vi "Main.vi"() -> ()   [LabVIEW 2022 SP3]
doc: "Main Program initialize config files, handles user inputs, image acquisition, object detection and image storing. User interface is handled in a state machine sending outputs."
uses:
  controls/State.ctl
  controls/Data.ctl
  <vilib>/userdefined/High Color/IMAQdx.ctl
  <vilib>/vision/Image Controls.llb/IMAQ Image.ctl
  b1a6e15a-21f6-4224-89c9-cebb1e441bce.vi
  4203ab90-da59-4329-829c-edbd02661f10.vi
  <extravilib>/ChannelInstances/Tag-bool/Read With Abort.vi
  <extravilib>/ChannelInstances/Tag-t'Data.ctl'/Read With Abort.vi
  <extravilib>/ChannelInstances/Tag-c(bool,bool)/Read With Abort.vi
  <extravilib>/ChannelInstances/Tag-c(bool,bool)/Write With Abort.vi
  <extravilib>/ChannelInstances/Tag-t'Data.ctl'/Write With Abort.vi
  <extravilib>/ChannelInstances/Tag-bool/Write With Abort.vi
  <extravilib>/ChannelInstances/Tag-c(bool,bool)/Instantiate.vi
  <extravilib>/ChannelInstances/Tag-t'Data.ctl'/Instantiate.vi
  <extravilib>/ChannelInstances/Tag-bool/Instantiate.vi
  <extravilib>/ChannelInstances/Tag-bool/EndpointRead.vi
  <extravilib>/ChannelInstances/Tag-t'Data.ctl'/EndpointRead.vi
  <extravilib>/ChannelInstances/Tag-c(bool,bool)/EndpointRead.vi
  <extravilib>/ChannelInstances/Tag-c(bool,bool)/Endpoint.vi
  <extravilib>/ChannelInstances/Tag-t'Data.ctl'/Endpoint.vi
  <extravilib>/ChannelInstances/Tag-bool/Endpoint.vi
  <extravilib>/ChannelInstances/Tag-bool.lvlib
  <extravilib>/ChannelInstances/Tag-t'Data.ctl'.lvlib
  <extravilib>/ChannelInstances/Tag-c(bool,bool).lvlib
panel:
  out "System Version":string="SRS Software - Version 0.0.0.1-beta"
  out "error out":errorcluster
  out "Overlay_tab":T1(tab)=enum."Connections"
  out "Cam1_Stats":cluster{"Mean_Area":i32, "Img_Count":u32} caption="Camera 1"
  out "Cam2_Stats":cluster{"Mean_Area":i32, "Img_Count":u32} caption="Camera 2"
  out "Sample Number":string="#0000" caption="Sample Name"
  in  "Collection Date":timestamp=timestamp(3501961200 s since 1904-01-01) format="%<%x>T"
  in  "Station":string="Station..." caption="Sample Name"
  in  "Location":string="Location..." caption="Sample Name"
  in  "Latitude":dbl caption="Sample Name" format="%.8g"
  in  "Longitude":dbl caption="Sample Name" format="%.8g"
  in  "Determiner":string="Name..." caption="Sample Name"
  in  "Sex":string="NaN" caption="Sample Name"
  in  "overloadThreshold":i32=5 caption="Overload threshold" min=1
  in  "saveQueueSize":i32=100 caption="Save Buffer Size" min=1
  in  "processQueueSize":i32=200 caption="Process Buffer Size" min=1
  in  "legacyAttributes":bool caption="Legacy Camera Attributes"
  in  "Change Crop":bool
  in  "DetectCrop":dbl=10.0 caption="Movement Detection size" format="%#_g %"
  in  "sampleSizeThreshold":i32=3000 caption="Sample size threshold" min=1
  in  "sampleTimeout":i32=20 caption="New Sample timeout" min=1
  out "Target framerate":i32=50 caption="Target FPS"
  in  "framerateMax":i32=50 caption="Max FPS" min=1
  in  "Exposure Time":dbl=2000.0
  in  "Exposure":enum32{"Item 0", "Item 1", "Item 2", "Item 3"}(radio)=enum."Item 3"
  in  "Aperture":enum32{"Item 0", "Item 1", "Item 2", "Item 3"}(radio)=enum."Item 1"
  in  "Calibration Pictures":bool
  in  "Empty Cuvette":bool
  in  "Manual Close":bool
  out "Current Position":string
  in  "Position":bool
  in  "flushSize":i32=150 caption="Flush Size" min=0 max=1000
  in  "dispenseDuration":i32=60 caption="Dispense Duration" min=20 max=200
  in  "Pump Cycle":bool
  in  "Pump Bottom":bool
  in  "Pump Top":bool
  in  "Pump Terminate":bool
  out "Process buffer":T2(graph)
  out "Save buffer":T2(graph)
  out "Framerate":i32 caption="Current Framerate"
  out "System Serial":string
  in  "Connect Systems":bool
  out "Actuator":bool
  out "Pump":bool
  out "Camera 1":bool
  out "Camera 2":bool
  in  "Override System":bool
  in  "Empty System":bool
  in  "Start System":bool
  out "Errors":errorcluster
  in  "Overlay_Ring":u16(ring)=6 items=["Session Data", "Extended Setup", "Buffer", "Camera", "Dispenser", "Stats", "Connections", "Errors"]
  in  "otherNotes":string caption="Other notes"
  in  "Species Name":string="System Test - Toke" caption="Sample Name"
  out "Ready":bool
  in  "Operator":string="MRJ" caption="Sample Name"
  out "Active":bool
  in  "Start Image Capture":bool
  in  "voucherId":string="#0000" caption="Voucher ID"
  in  "Stop Image Capture":bool
  in  "Empty and Refill":bool
  in  "Close and Refill":bool
  in  "Manual Open":bool
  out "Detection error":errorcluster
  out "Camera 1":T3(plugin-control)
  out "Camera 2":T3(plugin-control)
  out "Camera 1 Binary":T3(plugin-control)
  out "Camera 2 Binary":T3(plugin-control)
  out "Camera 1 Detect":T3(plugin-control)
  out "Camera 2 Detect":T3(plugin-control)
  # "Description:\nData from the last sample for each camera.\n\nMean area\nMean area  from detection algorithm.\n\nImages\nTotal number of images saved."
  # "Detection settings"
  # "Camera/Lens settings"
  # "Hatch Control"
  # "Pump Control"
  # "Connections"
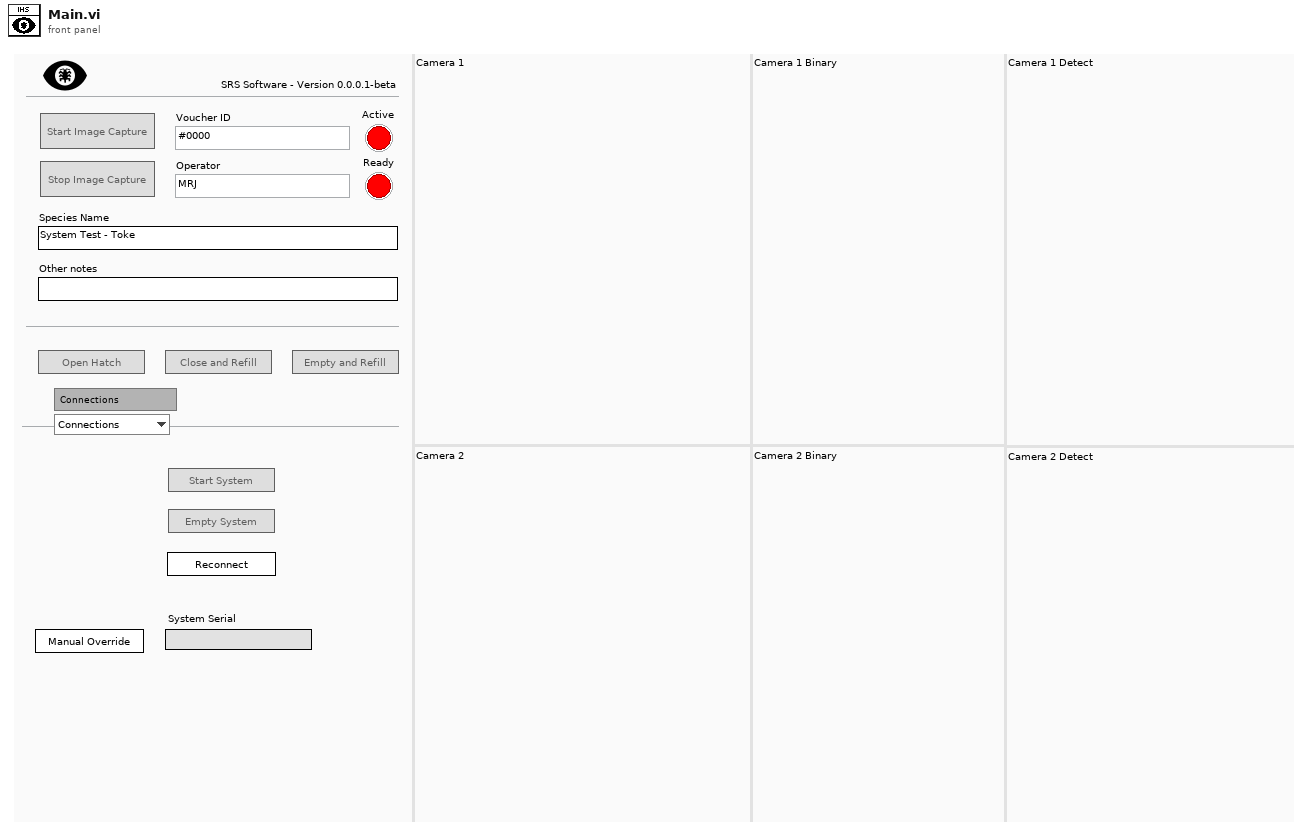
[diagram p1: front panel]
types:
  T1 = enum32{"Session Data", "Extended Setup", "Buffer", "Camera", "Dispenser", "Stats", "Connections", "Errors"}
  T2 = cluster{"# elements in queue":i32, "# elements in queue":i32}
  T3 = typedef "IMAQ Image.ctl" = refnum<image>
  T4 = typedef "Data.ctl" = cluster{"system":cluster{"info":cluster{"menuSelect":u16, "version":u16, "serial":string, "captureActive":bool, "captureBegin":bool, "emptyAndRefill":bool}, "userInfo":cluster{"operatorName":string, "date":timestamp}, "camera":cluster{"exposureTime":i32, "aperture":enum32{"Item 0", "Item 1", "Item 2", "Item 3"}, "framerate":i32, "framerateMax":i32, "legacyAttributes":bool}}, "connections":cluster{"arduino":cluster{"connection":refnum<visa-resource-name>, "status":bool, "openState":bool, "emptyStart":u32}, "pump":cluster{"connection":refnum<visa-resource-name>, "status":bool, "command":string, "dispenseSpeed":i32, "flushSize":i32}, "camera":cluster{"cam1":cluster{"connection":T5, "status":bool}, "cam2":cluster{"connection":T5, "status":bool}}}, "queue":cluster{"process":cluster{"cam1":refnum<queue>, "cam2":refnum<queue>, "queueSize":i32}, "save":cluster{"cam1":refnum<queue>, "cam2":refnum<queue>, "queueSize":i32}, "overloadThreshold":i32}, "imageProcess":cluster{"cam1":cluster{"preAllocation":cluster{"image":T3, "originalDisplay":T3, "originalRgb":T3, "binary":T3, "save":T3, "calibrationFull":T3, "calibrationDetect":T3}, "calibration":cluster{"pathFull":path, "pathDetect":path, "ROI":T6}}, "cam2":cluster{"preAllocation":cluster{"image":T3, "originalDisplay":T3, "originalRgb":T3, "binary":T3, "save":T3, "calibrationFull":T3, "calibrationDetect":T3}, "calibration":cluster{"pathFull":path, "pathDetect":path, "ROI":T6}}, "process":cluster{"planeExtract":T3, "planeSubtract":T3, "cropMask":T3}, "detection":cluster{"sampleTimeout":i32, "sizeThreshold":i32, "detectionRegionPct":dbl}}, "sampleData":cluster{"sampleId":string, "projectId":string, "voucherID":string, "speciesName":string, "collectionDate":timestamp, "sampleStation":string, "location":string, "lat":dbl, "lon":dbl, "determiner":string, "sex":string, "otherNotes":string}, "Session In":T5}
  T5 = typedef "IMAQdx.ctl" = refnum<k21>
  T6 = typedef "IMAQ Rectangle" = cluster{"Left":i32, "Top":i32, "Right":i32, "Bottom":i32, "Rotation":dbl}
  T7 = typedef "State.ctl" = enum16{"Initialize", "Wait for Event", "Position", "Valve Signal", "Extra Flush", "Valve Cycle", "Valve Open", "Valve Close", "Pump Command", "Pump Cycle", "Empty System", "Start System", "Connect Systems", "Start Image Capture", "Stop Image Capture", "Calibration Pictures", "Close and Refill", "Empty and Refill", "Change Light Intensity", "Reconnect", "CursorIdle", "Exit"}
  T8 = enum8{"Enabled", "Disabled", "Disabled and Grayed Out"}
  T9 = cluster{"# elements in queue":i32, "# elements in queue":i32}[]
  T10 = typedef "Tag-t'Data.ctl'.lvlib/))Channel.ctl" = refnum<queue>
  T11 = typedef "Tag-bool.lvlib/))Channel.ctl" = refnum<queue>
  T12 = typedef "Tag-c(bool,bool).lvlib/))Channel.ctl" = refnum<queue>
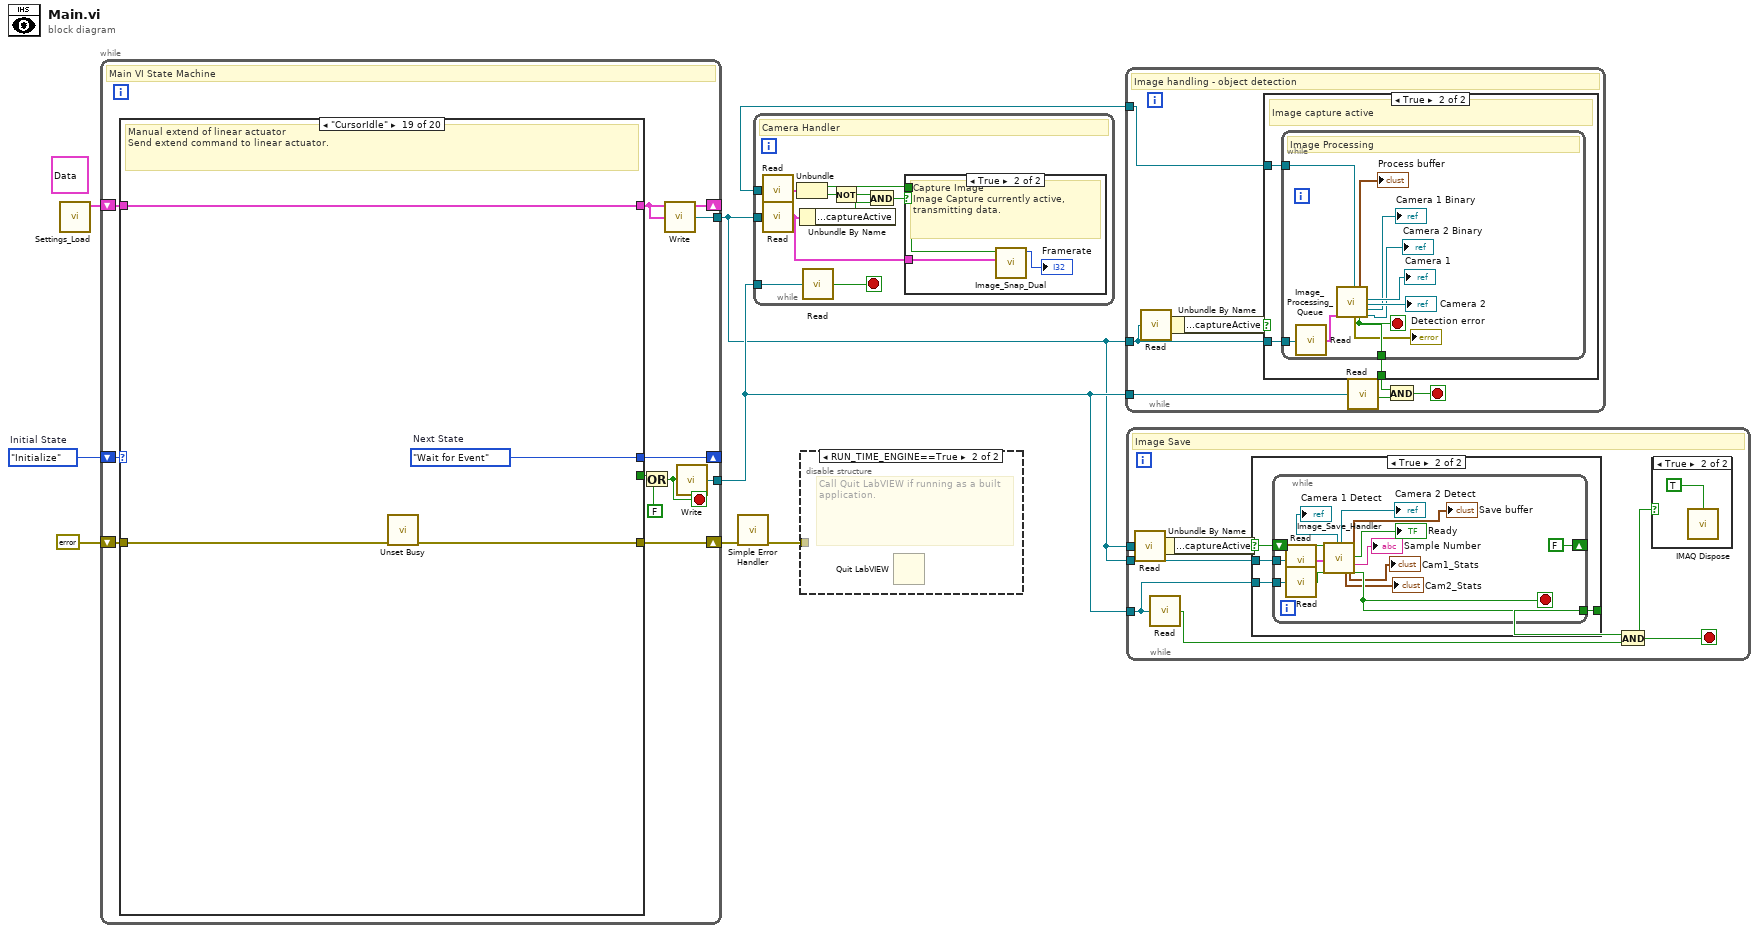
[diagram p0: block diagram]
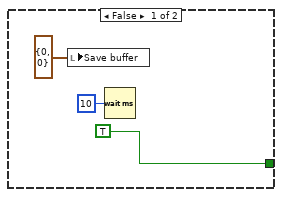
[diagram p3: hidden frame]
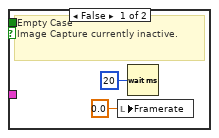
[diagram p4: hidden frame]
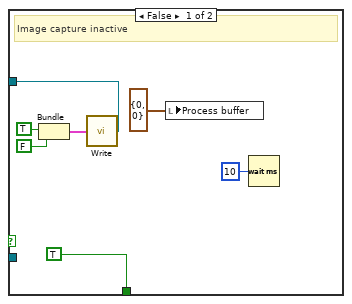
[diagram p5: hidden frame]
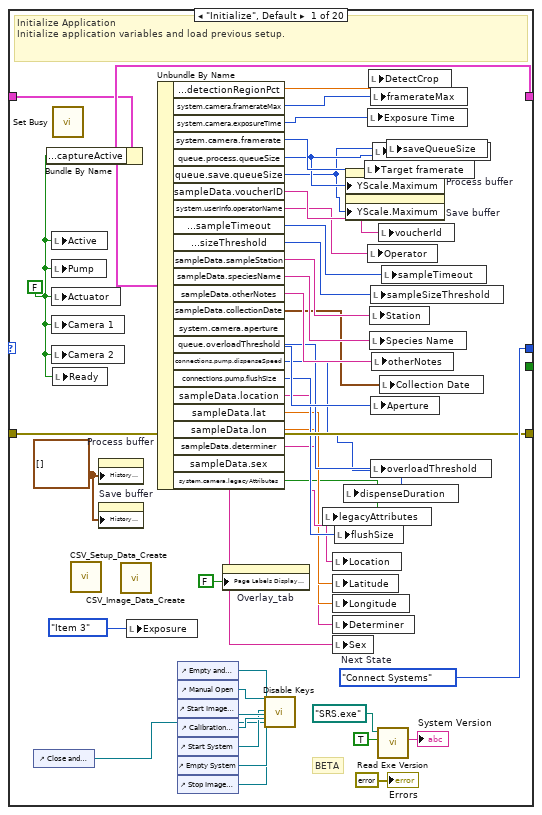
[diagram p7: hidden frame]
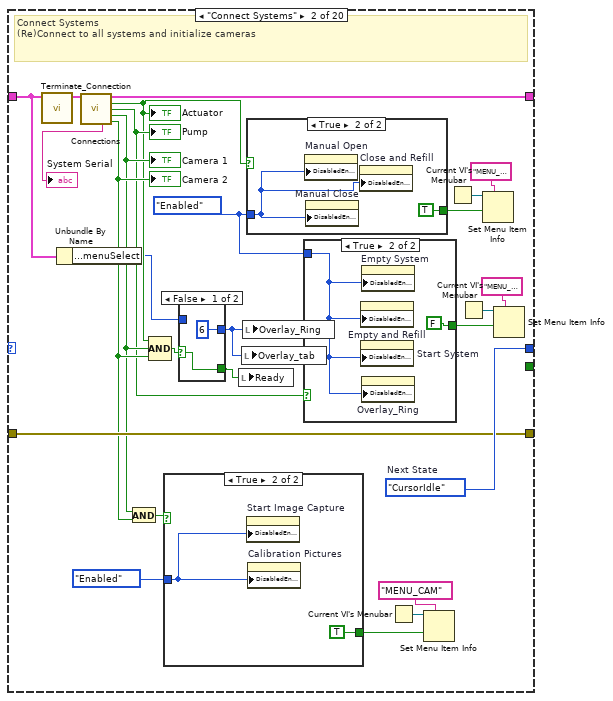
[diagram p8: hidden frame]
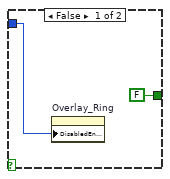
[diagram p10: hidden frame]
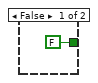
[diagram p11: hidden frame]
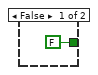
[diagram p12: hidden frame]
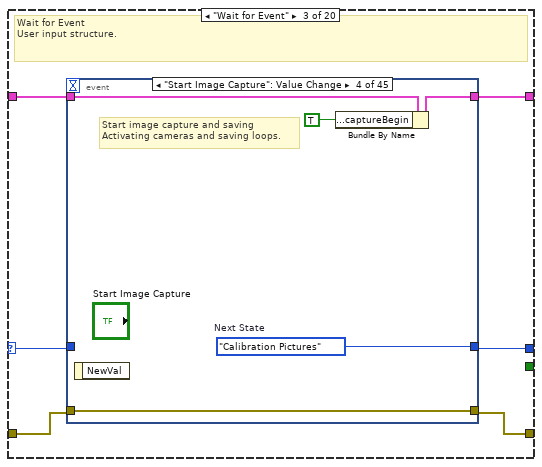
[diagram p13: hidden frame]
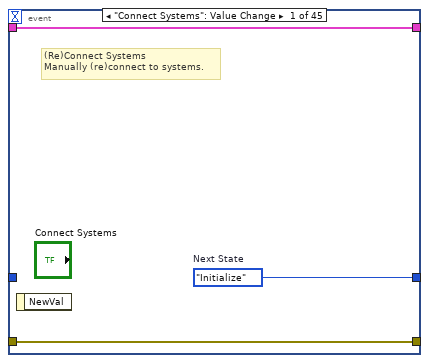
[diagram p14: hidden frame]
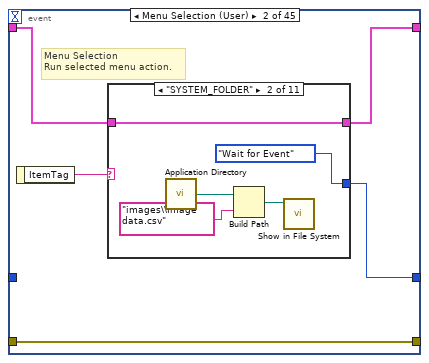
[diagram p15: hidden frame]
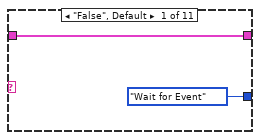
[diagram p16: hidden frame]
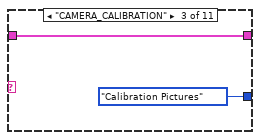
[diagram p17: hidden frame]
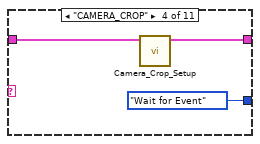
[diagram p18: hidden frame]
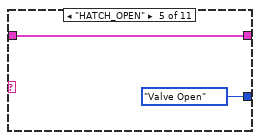
[diagram p19: hidden frame]
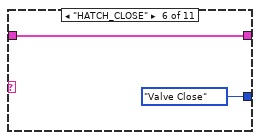
[diagram p20: hidden frame]
diagram:
  (unwired) T4 {"system"={"info"={"menuSelect"=0, "version"=0, "serial"="Test Sample", "captureActive"=FALSE, "captureBegin"=FALSE, "emptyAndRefill"=FALSE}, "userInfo"={"operatorName"="", "date"=timestamp(2713993200 s since 1904-01-01)}, "camera"={"exposureTime"=0, "aperture"=enum."Item 0", "framerate"=0, "framerateMax"=500, "legacyAttributes"=FALSE}}, "connections"={"arduino"={"connection"="", "status"=FALSE, "openState"=FALSE, "emptyStart"=0}, "pump"={"connection"="", "status"=FALSE, "command"="", "dispenseSpeed"=100, "flushSize"=100}, "camera"={"cam1"={"connection"="", "status"=FALSE}, "cam2"={"connection"="", "status"=FALSE}}}, "queue"={"process"={"cam1"=refnum, "cam2"=refnum, "queueSize"=0}, "save"={"cam1"=refnum, "cam2"=refnum, "queueSize"=0}, "overloadThreshold"=0}, "imageProcess"={"cam1"={"preAllocation"={"image"="Station", "originalDisplay"="Station", "originalRgb"="Station", "binary"="Station", "save"="Station", "calibrationFull"=refnum, "calibrationDetect"=refnum}, "calibration"={"pathFull"=path "C:/Users/au540322/Desktop/IHS_Project/images/Debris/Debris_0/Debris_0_2019_06_01-23-32-49-686.PNG", "pathDetect"=path "C:/Users/au540322/Desktop/IHS_Project/images/Debris/Debris_0/Debris_0_2019_06_01-23-32-49-686.PNG", "ROI"={"Left"=0, "Top"=0, "Right"=0, "Bottom"=0, "Rotation"=0.0}}}, "cam2"={"preAllocation"={"image"=refnum, "originalDisplay"=refnum, "originalRgb"=refnum, "binary"=refnum, "save"=refnum, "calibrationFull"=refnum, "calibrationDetect"=refnum}, "calibration"={"pathFull"=path "C:/Users/au540322/Desktop/IHS_Project/images/Debris/Debris_0/Debris_0_2019_06_01-23-32-49-686.PNG", "pathDetect"=path "C:/Users/au540322/Desktop/IHS_Project/images/Debris/Debris_0/Debris_0_2019_06_01-23-32-49-686.PNG", "ROI"={"Left"=0, "Top"=0, "Right"=0, "Bottom"=0, "Rotation"=0.0}}}, "process"={"planeExtract"=refnum, "planeSubtract"=refnum, "cropMask"=refnum}, "detection"={"sampleTimeout"=500, "sizeThreshold"=500, "detectionRegionPct"=0.0}}, "sampleData"={"sampleId"="", "projectId"="", "voucherID"="", "speciesName"="", "collectionDate"=timestamp(2713993200 s since 1904-01-01), "sampleStation"="", "location"="", "lat"=0.0, "lon"=0.0, "determiner"="", "sex"="", "otherNotes"=""}, "Session In"=""} ("Data")
  w8 = State."Initialize"  # Initial State
  n1 = call "Settings_Load.vi"() -> ("value"=w4:T4)  [unwired: 10 in, 1 out]
  n2 = while {
    shift-right: [w18] -> _
    shift-left: w8 -> [w19]
    shift-right: [w16] -> _
    shift-left: w4 -> [w17]
    shift-right: [w13] -> w6
    shift-left: errorcluster {"status"=FALSE, "code"=0, "source"=""} ("error constant") -> [w15]
    tunnel: [w10] -> w3
    tunnel: [w11] -> w2
    stop <- w14 stop-if-true
    # "Main VI State Machine"
    n3 = case shown="\"CursorIdle\"" w19 {
      selector: w19 -> [_ _ w104 _ _ _ _ _ _ _ _ _ _ _ _ _ _ _ _ _]
      tunnel: [w63 w89 w109 w376 w394 w413 w443 w468 w474 w491 w508 w516 w529 w547 w557 w587 w609 w627 w630 w641] -> w18
      tunnel: [_ _ _ _ _ _ _ _ _ _ _ _ _ _ _ _ _ _ _ w640] -> w12
      tunnel: w17 -> [w56 w69 w108 w377 w390 w406 w437 w462 w478 w495 w500 w514 w527 w546 w551 w586 w599 w611 w631 w636]
      tunnel: [w61 w87 w107 w378 w392 w405 w442 w467 w469 w495 w501 w511 w526 w546 w550 w586 w598 w610 w631 w638] -> w16
      tunnel: w15 -> [w62 w88 w106 w379 w393 w412 w432 w457 w477 w492 w506 w519 w531 w542 w554 w583 w606 w624 w629 w634]
      tunnel: [w62 w88 w105 w379 w393 w412 w426 w450 w477 w485 w505 w517 w520 w541 w553 w580 w605 w615 w628 w635] -> w13
      frame "Initialize", Default {
        w55 = T9 [] ("History Data")
        w54 = FALSE ("Pump")
        w63 = State."Connect Systems"  # Next State
        # "BETA"
        # "Initialize Application\nInitialize application variables and load previous setup."
        n4 = control-ref of="Close and Refill"() -> (w39:refnum<vi>)
        n5 = Bundle By Name(cluster=w56, "system.info.captureActive"=w54) -> (w61:T4)
        n6 = local write "Active"(w54) -> ()
        n7 = local write "Pump"(w54) -> ()
        n8 = local write "Actuator"(w54) -> ()
        n9 = local write "Camera 1"(w54) -> ()
        n10 = local write "Camera 2"(w54) -> ()
        n11 = call <vilib>:"Set Busy.vi"() -> ()  [unwired: 10 in, 2 out]
        n12 = local write "Ready"(w54) -> ()
        n13 = call "CSV_Setup_Data_Create.vi"() -> ()  [unwired: 11 in, 1 out]
        n14 = property on="Process buffer" class="WFChart (strict)"("History Data"=w55) -> ()  [unwired: 2 in, 2 out]
        n15 = property on="Save buffer" class="WFChart (strict)"("History Data"=w55) -> ()  [unwired: 2 in, 2 out]
        n16 = call "CSV_Image_Data_Create.vi"() -> ()  [unwired: 12 in]
        n17 = local write "Exposure"(enum32{"Item 0", "Item 1", "Item 2", "Item 3"}."Item 3" ("Exposure")) -> ()
        n18 = Unbundle By Name(w61) -> ("imageProcess.detection.detectionRegionPct"=w36:dbl, "system.camera.framerateMax"=w37:i32, "system.camera.exposureTime"=w60:i32, "system.camera.framerate"=w59:i32, "queue.process.queueSize"=w21:i32, "queue.save.queueSize"=w20:i32, "sampleData.voucherID"=w58:string, "system.userInfo.operatorName"=w57:string, "imageProcess.detection.sampleTimeout"=w53:i32, "imageProcess.detection.sizeThreshold"=w52:i32, "sampleData.sampleStation"=w51:string, "sampleData.speciesName"=w50:string, "sampleData.otherNotes"=w49:string, "sampleData.collectionDate"=w22:timestamp, "system.camera.aperture"=w48:enum32{"Item 0", "Item 1", "Item 2", "Item 3"}, "queue.overloadThreshold"=w47:i32, "connections.pump.dispenseSpeed"=w34:i32, "connections.pump.flushSize"=w35:i32, "sampleData.location"=w33:string, "sampleData.lat"=w32:dbl, "sampleData.lon"=w31:dbl, "sampleData.determiner"=w30:string, "sampleData.sex"=w29:string, "system.camera.legacyAttributes"=w28:bool)
        n19 = control-ref of="Empty and Refill"() -> (w46:refnum<vi>)
        n20 = control-ref of="Manual Open"() -> (w45:refnum<vi>)
        n21 = control-ref of="Start Image Capture"() -> (w43:refnum<vi>)
        n22 = control-ref of="Calibration Pictures"() -> (w44:refnum<vi>)
        n23 = control-ref of="Start System"() -> (w42:refnum<vi>)
        n24 = control-ref of="Empty System"() -> (w41:refnum<vi>)
        n25 = control-ref of="Stop Image Capture"() -> (w40:refnum<vi>)
        n26 = property on="Overlay_tab" class="TabCtl (strict)"("Page Labels Display Visible?"=FALSE) -> ()  [unwired: 2 in, 2 out]
        n27 = call "Disable Keys.vi"("Boolean in"=w45, "Bool Refnum 6"=w46, "Bool Refnum 4"=w40, "Bool Refnum 7"=w42, "Bool Refnum 9"=w43, "Bool Refnum 2"=w44, "Bool Refnum 8"=w39, "Bool Refnum 3"=w41) -> ()  [unwired: 20 in]
        n28 = local write "legacyAttributes"(w28) -> ()
        n29 = local write "Location"(w33) -> ()
        n30 = local write "Latitude"(w32) -> ()
        n31 = local write "Longitude"(w31) -> ()
        n32 = local write "Determiner"(w30) -> ()
        n33 = local write "Sex"(w29) -> ()
        n34 = local write "flushSize"(w35) -> ()
        n35 = local write "dispenseDuration"(w34) -> ()
        n36 = property on="Process buffer" class="WFChart (strict)"("YScale.Maximum"=w21) -> ()  [unwired: 2 in, 2 out]
        n37 = property on="Save buffer" class="WFChart (strict)"("YScale.Maximum"=w20) -> ()  [unwired: 2 in, 2 out]
        n38 = local write "Target framerate"(w59) -> ()
        n39 = local write "Exposure Time"(w60) -> ()
        n40 = local write "Operator"(w57) -> ()
        n41 = local write "DetectCrop"(w36) -> ()
        n42 = local write "Station"(w51) -> ()
        n43 = local write "Species Name"(w50) -> ()
        n44 = local write "framerateMax"(w37) -> ()
        n45 = local write "sampleSizeThreshold"(w52) -> ()
        n46 = local write "Aperture"(w48) -> ()
        n47 = local write "overloadThreshold"(w47) -> ()
        n48 = local write "otherNotes"(w49) -> ()
        n49 = local write "processQueueSize"(w21) -> ()
        n50 = call "Read Exe Version.vi"("beta?"=TRUE, "Application name"=path "SRS.exe") -> ("Title String"=→"System Version":string)  [unwired: 6 in, 3 out]
        n51 = local write "voucherId"(w58) -> ()
        n52 = local write "Collection Date"(w22) -> ()
        n53 = local write "sampleTimeout"(w53) -> ()
        n54 = local write "saveQueueSize"(w20) -> ()
        "Errors" <- errorcluster {"status"=FALSE, "code"=0, "source"=""} ("Calibration Error")
      }
      frame "Connect Systems" {
        w83 = T8."Enabled" ("Disabled")
        w89 = State."CursorIdle"  # Next State
        # "Connect Systems\n(Re)Connect to all systems and initialize cameras"
        n55 = call "Terminate_Connection.vi"("Data"=w69) -> ("Data out"=w86:T4)  [unwired: 9 in, 1 out]
        n56 = Unbundle By Name(w69) -> ("system.info.menuSelect"=w68:u16)
        n57 = call "Connections.vi"("input cluster"=w86) -> ("output cluster"=w87:T4, "Linear Actuator"=w70:bool, "Pump"=w71:bool, "Camear 1"=w72:bool, "System Serial"=→"System Serial":string, "Camera 2"=w73:bool)  [unwired: 9 in]
        "Pump" <- w71
        "Actuator" <- w70
        "Camera 2" <- w73
        "Camera 1" <- w72
        n58 = And(x=w72, y=w73) -> (x .and. y?=w85:bool)
        n59 = Compound Arithmetic op=AND(w70, w72, w73) -> (w67:bool)
        n60 = case shown="True" w85 {
          tunnel: T8."Enabled" ("Disabled") -> [_ w100]
          tunnel: [FALSE ("enabled") TRUE ("enabled")] -> w80
          frame False {
          }
          frame True {
            n61 = property on="Start Image Capture" class="Bool"("DisabledEnum"=w100) -> ()  [unwired: 2 in, 2 out]
            n62 = property on="Calibration Pictures" class="Bool"("DisabledEnum"=w100) -> ()  [unwired: 2 in, 2 out]
          }
        }
        n63 = case shown="False" w67 {
          selector: w67 -> [w90 w92]
          tunnel: w68 -> [_ w93]
          tunnel: [u16 6 ("Overlay_Ring") w93] -> w66
          tunnel: [w90 w92] -> w65
          frame False {
          }
          frame True {
          }
        }
        n64 = local write "Ready"(w65) -> ()
        n65 = local write "Overlay_tab"(w66) -> ()
        n66 = local write "Overlay_Ring"(w66) -> ()
        n67 = case shown="True" w70 {
          tunnel: w83 -> [_ w103]
          tunnel: [FALSE ("enabled") TRUE ("enabled")] -> w77
          frame False {
          }
          frame True {
            n68 = property on="Manual Open" class="Bool"("DisabledEnum"=w103) -> ()  [unwired: 2 in, 2 out]
            n69 = property on="Manual Close" class="Bool"("DisabledEnum"=w103) -> ()  [unwired: 2 in, 2 out]
            n70 = property on="Close and Refill" class="Bool"("DisabledEnum"=w103) -> ()  [unwired: 2 in, 2 out]
          }
        }
        n71 = case shown="True" w71 {
          tunnel: w83 -> [w95 w97]
          tunnel: [FALSE ("enabled") FALSE ("enabled")] -> w74
          frame False {
            n72 = property on="Overlay_Ring" class="Ring (strict)"("DisabledEnum"=w95) -> ()  [unwired: 2 in, 2 out]
          }
          frame True {
            n73 = property on="Empty and Refill" class="Bool"("DisabledEnum"=w97) -> ()  [unwired: 2 in, 2 out]
            n74 = property on="Start System" class="Bool"("DisabledEnum"=w97) -> ()  [unwired: 2 in, 2 out]
            n75 = property on="Empty System" class="Bool"("DisabledEnum"=w97) -> ()  [unwired: 2 in, 2 out]
            n76 = property on="Overlay_Ring" class="Ring (strict)"("DisabledEnum"=w97) -> ()  [unwired: 2 in, 2 out]
          }
        }
        n77 = Current VI's Menubar() -> (w82:refnum<k9>)
        n78 = Set Menu Item Info(7:"MENU_CAM" ("item tag"), 9:w80, 11:w82) -> ()  [unwired: 4 in, 2 out]
        n79 = Current VI's Menubar() -> (w78:refnum<k9>)
        n80 = Current VI's Menubar() -> (w76:refnum<k9>)
        n81 = Set Menu Item Info(7:"MENU_HATCH" ("item tag"), 9:w77, 11:w78) -> ()  [unwired: 4 in, 2 out]
        n82 = Set Menu Item Info(7:"MENU_HATCH" ("item tag"), 9:w74, 11:w76) -> ()  [unwired: 4 in, 2 out]
      }
      frame "Wait for Event" {
        # "Wait for Event\nUser input structure."
        n83 = event shown="[3] \"Start Image Capture\": Value Change" {
          selector: _ -> [_ _ _ _ _ _ _ _ _ _ _ _ _ _ _ _ _ _ _ _ _ _ _ _ _ _ _ _ _ _ _ _ _ _ _ _ _ _ _ _ _ _ _ _ _]
          dyn-events: _ -> [_ _ _ _ _ _ _ _ _ _ _ _ _ _ _ _ _ _ _ _ _ _ _ _ _ _ _ _ _ _ _ _ _ _ _ _ _ _ _ _ _ _ _ _ _]
          timeout: _ -> [_ _ _ _ _ _ _ _ _ _ _ _ _ _ _ _ _ _ _ _ _ _ _ _ _ _ _ _ _ _ _ _ _ _ _ _ _ _ _ _ _ _ _ _ _]
          tunnel: [w112 w115 w155 w160 w163 w166 w169 w172 w175 w178 w189 w192 w195 w198 w201 w204 w209 w214 w219 w220 w225 State."Wait for Event" ("Next State") State."Wait for Event" ("Next State") State."Wait for Event" ("Next State") State."Wait for Event" ("Next State") State."Wait for Event" ("Next State") State."Wait for Event" ("Next State") State."Wait for Event" ("Next State") State."Wait for Event" ("Next State") State."Wait for Event" ("Next State") State."Wait for Event" ("Next State") State."Wait for Event" ("Next State") State."Wait for Event" ("Next State") State."Wait for Event" ("Next State") w317 w322 w327 w332 w337 w347 w351 w356 State."Wait for Event" ("Next State") w368 w373] -> w109
          tunnel: w108 -> [w110 w114 w154 w158 w161 w164 w167 w170 w173 w176 w187 w190 w193 w196 w199 w202 w206 w211 w216 w223 w226 w231 w236 w241 w246 w251 w256 w261 w266 w271 w276 w283 w288 w311 w318 w323 w328 w333 w338 w342 w353 w358 w363 w366 w370]
          tunnel: [w110 w113 w154 w157 w161 w164 w167 w170 w173 w176 w187 w190 w193 w196 w199 w202 w205 w210 w215 w222 w227 w232 w237 w242 w247 w252 w257 w262 w267 w272 w277 w280 w296 w312 w319 w324 w329 w334 w339 w348 w352 w357 w362 w365 w370] -> w107
          tunnel: w106 -> [w111 w117 w153 w159 w162 w165 w168 w171 w174 w177 w188 w191 w194 w197 w200 w203 w208 w213 w218 w224 w229 w234 w239 w244 w249 w254 w259 w264 w269 w274 w279 w285 w298 w315 w320 w325 w330 w335 w340 w349 w354 w359 w364 w367 w372]
          tunnel: [w111 w117 w153 w159 w162 w165 w168 w171 w174 w177 w188 w191 w194 w197 w200 w203 w208 w213 w218 w224 w229 w234 w239 w244 w249 w254 w259 w264 w269 w274 w279 w285 w298 w315 w320 w325 w330 w335 w340 w349 w354 w359 w364 w367 w372] -> w105
          tunnel: w104 -> [_ _ _ _ _ _ _ _ _ _ _ _ _ _ _ _ _ _ _ _ _ _ _ _ _ _ _ _ _ _ _ _ _ _ _ _ _ _ _ _ _ _ _ _ _]
          event "Connect Systems": Value Change {
            w112 = State."Initialize"  # Next State
            # "(Re)Connect Systems\nManually (re)connect to systems."
            n84 = event-data() -> ()  [unwired: 1 in, 1 out]
          }
          event Menu Selection (User) {
            # "Menu Selection\nRun selected menu action."
            n85 = event-data() -> ("ItemTag"=w116:string)  [unwired: 1 in]
            n86 = case shown="\"SYSTEM_FOLDER\"" w116 {
              tunnel: [State."Wait for Event" ("Next State") State."Wait for Event" ("Next State") State."Calibration Pictures" ("Next State") State."Wait for Event" ("Next State") State."Valve Open" ("Next State") State."Valve Close" ("Next State") State."Start System" ("Next State") State."Empty System" ("Next State") State."Exit" ("Next State") State."Initialize" ("Next State") State."Wait for Event" ("Next State")] -> w115
              tunnel: w114 -> [w118 w123 w125 w128 w130 w133 w135 w137 w139 w141 w151]
              tunnel: [w118 w123 w125 w127 w130 w133 w135 w137 w139 w141 w151] -> w113
              frame "False", Default {
              }
              frame "SYSTEM_FOLDER" {
                n87 = call <vilib>:"Application Directory.vi"() -> ("Application Directory"=w122:path)
                n88 = Build Path(base path=w122, name or relative path="images\\Image data.csv" ("string")) -> (appended path=w120:path)
                n89 = call <vilib>:"Show in File System.vi"("file or directory path"=w120) -> ()  [unwired: 10 in, 1 out]
              }
              frame "CAMERA_CALIBRATION" {
              }
              frame "CAMERA_CROP" {
                n90 = call "Camera_Crop_Setup.vi"("value"=w128) -> ("output cluster"=w127:T4)  [unwired: 10 in]
              }
              frame "HATCH_OPEN" {
              }
              frame "HATCH_CLOSE" {
              }
              frame "SYSTEM_START" {
              }
              frame "SYSTEM_STOP" {
              }
              frame "SYS_EXIT" {
              }
              frame "SYSTEM_RECONNECT" {
              }
              frame "SYSTEM_OVERRIDE" {
                n91 = control-ref of="Empty and Refill"() -> (w142:refnum<vi>)
                n92 = control-ref of="Start Image Capture"() -> (w144:refnum<vi>)
                n93 = control-ref of="Manual Open"() -> (w145:refnum<vi>)
                n94 = control-ref of="Manual Open"() -> (w146:refnum<vi>)
                n95 = control-ref of="Calibration Pictures"() -> (w147:refnum<vi>)
                n96 = control-ref of="Empty System"() -> (w148:refnum<vi>)
                n97 = control-ref of="Start System"() -> (w149:refnum<vi>)
                n98 = control-ref of="Stop Image Capture"() -> (w150:refnum<vi>)
                n99 = call "Enable Keys.vi"("Boolean in"=w142, "Bool Refnum 2"=w144, "Bool Refnum 3"=w145, "Bool Refnum 4"=w146, "Bool Refnum 6"=w147, "Bool Refnum 7"=w148, "Bool Refnum 8"=w149, "Bool Refnum 9"=w150) -> ()  [unwired: 20 in]
              }
            }
          }
          event Panel Close? {
            w155 = State."Exit"  # Next State
            # "Exit program\nTerminates connections and memory\nallocations in Exit state and exit program."
            n100 = event-data() -> ()  [unwired: 1 in, 1 out]
            n101 = event-data("Discard?"=TRUE) -> ()  [unwired: 1 in, 1 out]
          }
          event "Start Image Capture": Value Change {
            w160 = State."Calibration Pictures"  # Next State
            # "Start image capture and saving\nActivating cameras and saving loops."
            n102 = event-data() -> ()  [unwired: 1 in, 1 out]
            n103 = Bundle By Name(cluster=w158, "system.info.captureBegin"=TRUE ("Img_Capt Begin")) -> (w157:T4)
          }
          event "Stop Image Capture": Value Change {
            w163 = State."Stop Image Capture"  # Next State
            # "Stop image capture and saving\nStops cameras and saving loops."
            n104 = event-data() -> ()  [unwired: 1 in, 1 out]
          }
          event "Calibration Pictures": Value Change {
            w166 = State."Calibration Pictures"  # Next State
            # "Start image capture and saving\nActivating cameras and saving loops."
            n105 = event-data() -> ()  [unwired: 1 in, 1 out]
          }
          event "Start System": Value Change {
            w169 = State."Start System"  # Next State
            # "Initialize Pump\nRun initialization of pump."
            n106 = event-data() -> ()  [unwired: 1 in, 1 out]
          }
          event "Empty System": Value Change {
            w172 = State."Empty System"  # Next State
            # "Empty system\nEmpty the pump and pipes."
            n107 = event-data() -> ()  [unwired: 1 in, 1 out]
          }
          event "Empty and Refill": Value Change {
            w175 = State."Empty and Refill"  # Next State
            # "Manually start empty and refill procedure\nRetracting actuator and start \nlistening for DONE signal."
            n108 = event-data() -> ()  [unwired: 1 in, 1 out]
          }
          event "Close and Refill": Value Change {
            w178 = State."Close and Refill"  # Next State
            # "Manually start empty and refill procedure\nRetracting actuator and start \nlistening for DONE signal."
            n109 = event-data() -> ()  [unwired: 1 in, 1 out]
          }
          event "Override System": Value Change {
            w189 = State."Wait for Event"  # Next State
            # "Override System\nAllowing full access to systems"
            n110 = event-data() -> ()  [unwired: 1 in, 1 out]
            n111 = control-ref of="Empty and Refill"() -> (w179:refnum<vi>)
            n112 = control-ref of="Start Image Capture"() -> (w180:refnum<vi>)
            n113 = control-ref of="Manual Open"() -> (w181:refnum<vi>)
            n114 = control-ref of="Manual Open"() -> (w182:refnum<vi>)
            n115 = control-ref of="Calibration Pictures"() -> (w183:refnum<vi>)
            n116 = control-ref of="Empty System"() -> (w184:refnum<vi>)
            n117 = control-ref of="Start System"() -> (w185:refnum<vi>)
            n118 = control-ref of="Stop Image Capture"() -> (w186:refnum<vi>)
            n119 = call "Enable Keys.vi"("Boolean in"=w179, "Bool Refnum 2"=w180, "Bool Refnum 3"=w181, "Bool Refnum 4"=w182, "Bool Refnum 6"=w183, "Bool Refnum 7"=w184, "Bool Refnum 8"=w185, "Bool Refnum 9"=w186) -> ()  [unwired: 20 in]
          }
          event "Empty Cuvette": Value Change {
            w192 = State."Valve Cycle"  # Next State
            # "Manual cycle of linear actuator\nRetract and extends linear actuator."
            n120 = event-data() -> ()  [unwired: 1 in, 1 out]
          }
          event "Manual Open": Value Change {
            w195 = State."Valve Open"  # Next State
            # "Manual extend\nManually extend linear actuator."
            n121 = event-data() -> ()  [unwired: 1 in, 1 out]
          }
          event "Manual Close": Value Change {
            w198 = State."Valve Close"  # Next State
            # "Manual Retract\nManually retract linear actuator."
            n122 = event-data() -> ()  [unwired: 1 in, 1 out]
          }
          event "Position": Value Change {
            w201 = State."Position"  # Next State
            # "Read position\nRead linear actuator position."
            n123 = event-data() -> ()  [unwired: 1 in, 1 out]
          }
          event "Pump Cycle": Value Change {
            w204 = State."Pump Cycle"  # Next State
            # "Manual Pump Cycle\nManually go through a pump cycle."
            n124 = event-data() -> ()  [unwired: 1 in, 1 out]
          }
          event "Pump Top": Value Change {
            w209 = State."Pump Command"  # Next State
            # "Manual Move Pump Top\nManually move the pump \nto the top position."
            n125 = event-data() -> ()  [unwired: 1 in, 1 out]
            n126 = Bundle By Name(cluster=w206, "connections.pump.command"="A1000R" ("write buffer 2")) -> (w205:T4)
          }
          event "Pump Bottom": Value Change {
            w214 = State."Pump Command"  # Next State
            # "Manual Move Pump Bottom\nManually move the pump\nto the bottom position."
            n127 = event-data() -> ()  [unwired: 1 in, 1 out]
            n128 = Bundle By Name(cluster=w211, "connections.pump.command"="A0R" ("write buffer 2")) -> (w210:T4)
          }
          event "Pump Terminate": Value Change {
            w219 = State."Pump Command"  # Next State
            # "Terminate Pump\nAbort all current pump commands, \nacts as emergency stop."
            n129 = event-data() -> ()  [unwired: 1 in, 1 out]
            n130 = Bundle By Name(cluster=w216, "connections.pump.command"="T" ("write buffer 2")) -> (w215:T4)
          }
          event "voucherId": Value Change {
            w220 = State."Wait for Event"  # Next State
            # "Sample Name\nSample Name, used in image folders,\nand saved in sample information file."
            n131 = event-data() -> ()  [unwired: 1 in, 3 out]
            n132 = Bundle By Name(cluster=w223, "sampleData.projectId"="voucherId") -> (w222:T4)
          }
          event "Operator": Value Change {
            w225 = State."Wait for Event"  # Next State
            # "Operator Name\nOperator Name, saved in sample information file."
            n133 = event-data() -> ()  [unwired: 1 in, 3 out]
            n134 = Bundle By Name(cluster=w226, "system.userInfo.operatorName"="Operator") -> (w227:T4)
          }
          event "Species Name": Value Change {
            # "Sample Notes\nNotes/Description, saved in sample \ninformation file."
            n135 = event-data() -> ()  [unwired: 1 in, 3 out]
            n136 = Bundle By Name(cluster=w231, "sampleData.speciesName"="Species Name") -> (w232:T4)
          }
          event "Collection Date": Value Change {
            # "Collection Date\nSample collection date, saved in sample \ninformation file."
            n137 = event-data() -> ()  [unwired: 1 in, 3 out]
            n138 = Bundle By Name(cluster=w236, "sampleData.collectionDate"="Collection Date") -> (w237:T4)
          }
          event "Station": Value Change {
            # "Sample Notes\nNotes/Description, saved in sample \ninformation file."
            n139 = event-data() -> ()  [unwired: 1 in, 3 out]
            n140 = Bundle By Name(cluster=w241, "sampleData.sampleStation"="Station") -> (w242:T4)
          }
          event "Location": Value Change {
            # "Location\nNotes/Description, saved in sample \ninformation file."
            n141 = event-data() -> ()  [unwired: 1 in, 3 out]
            n142 = Bundle By Name(cluster=w246, "sampleData.location"="Location") -> (w247:T4)
          }
          event "Latitude": Value Change {
            # "Latitude\nNotes/Description, saved in sample \ninformation file."
            n143 = event-data() -> ()  [unwired: 1 in, 3 out]
            n144 = Bundle By Name(cluster=w251, "sampleData.lat"="Latitude") -> (w252:T4)
          }
          event "Longitude": Value Change {
            # "Longitude\nNotes/Description, saved in sample \ninformation file."
            n145 = event-data() -> ()  [unwired: 1 in, 3 out]
            n146 = Bundle By Name(cluster=w256, "sampleData.lon"="Longitude") -> (w257:T4)
          }
          event "Determiner": Value Change {
            # "Determiner\nNotes/Description, saved in sample \ninformation file."
            n147 = event-data() -> ()  [unwired: 1 in, 3 out]
            n148 = Bundle By Name(cluster=w261, "sampleData.determiner"="Determiner") -> (w262:T4)
          }
          event "Sex": Value Change {
            # "Sex\nNotes/Description, saved in sample \ninformation file."
            n149 = event-data() -> ()  [unwired: 1 in, 3 out]
            n150 = Bundle By Name(cluster=w266, "sampleData.sex"="Sex") -> (w267:T4)
          }
          event "legacyAttributes": Value Change {
            # "Legacy Camera Attributes\nEnable/Disable Legacy Camera Attributes."
            n151 = event-data() -> ()  [unwired: 1 in, 3 out]
            n152 = Bundle By Name(cluster=w271, "system.camera.legacyAttributes"="legacyAttributes") -> (w272:T4)
          }
          event "otherNotes": Value Change {
            # "Sample Notes\nNotes/Description, saved in sample \ninformation file."
            n153 = event-data() -> ()  [unwired: 1 in, 3 out]
            n154 = Bundle By Name(cluster=w276, "sampleData.otherNotes"="otherNotes") -> (w277:T4)
          }
          event "Aperture": Value Change {
            # "Aperture\nAperture setting (manually changed on cameras)\nsaved in information file. Loads calibration image."
            n155 = event-data() -> ()  [unwired: 1 in, 3 out]
            n156 = Bundle By Name(cluster=w283, "system.camera.aperture"="Aperture") -> (w281:T4)
            n157 = call "Calibration_Update.vi"("value"=w281) -> ("output cluster"=w280:T4)  [unwired: 10 in]
          }
          event "Exposure": Value Change {
            n158 = event-data() -> ()  [unwired: 1 in, 3 out]
            n159 = Unbundle By Name(w288) -> ("system.camera.framerateMax"=w293:i32)
            n160 = case shown="\"Item 3\"" "Exposure" {
              tunnel: [1000.0 1500.0 2000.0 w302] -> w286
              frame "Item 0", Default {
              }
              frame "Item 1" {
              }
              frame "Item 2" {
              }
              frame "Item 3" {
                n161 = local read "Exposure Time"() -> (w302:dbl)
              }
            }
            n162 = Multiply(x=w286, y=10.0) -> (x*y=w291:dbl)
            n163 = Divide(x=1000000.0, y=w291) -> (x/y=w292:dbl)
            n164 = Max & Min(x=w292, y=w293) -> (min(x,y)=w294:dbl)  [unwired: 1 out]
            n165 = local write "Exposure Time"(w286) -> ()
            n166 = Bundle By Name(cluster=w288, "system.camera.exposureTime"=w286, "system.camera.framerate"=w294) -> (w287:T4)
            n167 = local write "Target framerate"(w294) -> ()
            n168 = call "Calibration_Update.vi"("value"=w287) -> ("output cluster"=w296:T4)  [unwired: 10 in]
          }
          event "Exposure Time": Value Change {
            # "Exposure Time\nChanges camera exposure time, must restart image\nacquisition to enable new value. Value is saved in \nsample information file."
            n169 = event-data() -> ()  [unwired: 1 in, 3 out]
            n170 = Unbundle By Name(w311) -> ("system.camera.framerateMax"=w305:i32)
            n171 = Multiply(x="Exposure Time", y=10.0) -> (x*y=w308:dbl)
            n172 = Divide(x=1000000.0, y=w308) -> (x/y=w306:dbl)
            n173 = Max & Min(x=w306, y=w305) -> (min(x,y)=w304:dbl)  [unwired: 1 out]
            "Target framerate" <- w304
            n174 = Bundle By Name(cluster=w311, "system.camera.exposureTime"="Exposure Time", "system.camera.framerate"=w304) -> (w313:T4)
            n175 = local write "Exposure"(enum32{"Item 0", "Item 1", "Item 2", "Item 3"}."Item 3" ("Exposure")) -> ()
            n176 = call "Calibration_Update.vi"("value"=w313) -> ("output cluster"=w312:T4)  [unwired: 10 in]
          }
          event "processQueueSize": Value Change {
            w317 = State."Wait for Event"  # Next State
            # "Image Processing Queue Size\nMaximum buffer size of the image processing queue."
            n177 = event-data() -> ()  [unwired: 1 in, 3 out]
            n178 = Bundle By Name(cluster=w318, "queue.process.queueSize"="processQueueSize") -> (w319:T4)
            n179 = property on="Process buffer" class="WFChart (strict)"("YScale.Maximum"="processQueueSize") -> ()  [unwired: 2 in, 2 out]
          }
          event "saveQueueSize": Value Change {
            w322 = State."Wait for Event"  # Next State
            # "Image Save Queue Size\nMaximum buffer size of the image saving queue."
            n180 = event-data() -> ()  [unwired: 1 in, 3 out]
            n181 = Bundle By Name(cluster=w323, "queue.save.queueSize"="saveQueueSize") -> (w324:T4)
            n182 = property on="Save buffer" class="WFChart (strict)"("YScale.Maximum"="saveQueueSize") -> ()  [unwired: 2 in, 2 out]
          }
          event "overloadThreshold": Value Change {
            w327 = State."Wait for Event"  # Next State
            # "Overload threshold (Image Processing)\nSet buffer size limit to overloading threshold. Values over this\nthreshold (while no object currently detected), will pause image\ncapture until image processing queue is empty."
            n183 = event-data() -> ()  [unwired: 1 in, 3 out]
            n184 = Bundle By Name(cluster=w328, "queue.overloadThreshold"="overloadThreshold") -> (w329:T4)
          }
          event "dispenseDuration": Value Change {
            w332 = State."Wait for Event"  # Next State
            # "Dispense Duration (Pump speed)\nDescription..."
            n185 = event-data() -> ()  [unwired: 1 in, 3 out]
            n186 = Bundle By Name(cluster=w333, "connections.pump.dispenseSpeed"="dispenseDuration") -> (w334:T4)
          }
          event "flushSize": Value Change {
            w337 = State."Wait for Event"  # Next State
            # "Flush Size (Extra flush)\nDescription..."
            n187 = event-data() -> ()  [unwired: 1 in, 3 out]
            n188 = Bundle By Name(cluster=w338, "connections.pump.flushSize"="flushSize") -> (w339:T4)
          }
          event "framerateMax": Value Change {
            w347 = State."Wait for Event"  # Next State
            # "Maximum Framerate\nMaximum image capture framerate."
            n189 = event-data() -> ()  [unwired: 1 in, 3 out]
            n190 = Unbundle By Name(w342) -> ("system.camera.exposureTime"=w345:i32)
            n191 = Divide(x=10000000, y=w345) -> (x/y=w346:dbl)
            n192 = Max & Min(x="framerateMax", y=w346) -> (min(x,y)=w341:dbl)  [unwired: 1 out]
            n193 = Bundle By Name(cluster=w342, "system.camera.framerateMax"="framerateMax", "system.camera.framerate"=w341) -> (w348:T4)
            n194 = local write "Target framerate"(w341) -> ()
          }
          event "sampleTimeout": Value Change {
            w351 = State."Wait for Event"  # Next State
            # "Sample Timeout\nDefined the timeout duration used to determine a new sample."
            n195 = event-data() -> ()  [unwired: 1 in, 3 out]
            n196 = Bundle By Name(cluster=w353, "imageProcess.detection.sampleTimeout"="sampleTimeout") -> (w352:T4)
          }
          event "sampleSizeThreshold": Value Change {
            w356 = State."Wait for Event"  # Next State
            # "Framerate\nDefined the save frequency (saves every nth image)\nValue saved in sample information file."
            n197 = event-data() -> ()  [unwired: 1 in, 3 out]
            n198 = Bundle By Name(cluster=w358, "imageProcess.detection.sizeThreshold"="sampleSizeThreshold") -> (w357:T4)
          }
          event "DetectCrop": Value Change {
            # "Movement Detection Crop %\nChanges the percentage of the image used for detecting\nmovement, before full image is tracked."
            n199 = event-data() -> ()  [unwired: 1 in, 3 out]
            n200 = Bundle By Name(cluster=w363, "imageProcess.detection.detectionRegionPct"="DetectCrop") -> (w362:T4)
          }
          event "Change Crop": Value Change {
            w368 = State."Wait for Event"  # Next State
            # "Change crop\nChange the cropping of images."
            n201 = event-data() -> ()  [unwired: 1 in, 1 out]
            n202 = call "Camera_Crop_Setup.vi"("value"=w366) -> ("output cluster"=w365:T4)  [unwired: 10 in]
          }
          event "Overlay_Ring": Value Change {
            w373 = State."Wait for Event"  # Next State
            # "Change Overlay\nChange the main screen overlay."
            n203 = event-data() -> ()  [unwired: 1 in, 1 out]
            n204 = property on="Overlay_Ring" class="Ring (strict)"("Key Focus"=TRUE) -> ()  [unwired: 2 in, 2 out]
            "Overlay_tab" <- "Overlay_Ring"
          }
        }
      }
      frame "Start Image Capture" {
        # "Start Image Capture\nActivating Camera and Image saving loops."
        n205 = call "Calibration_Load.vi"("Data in"=w377) -> ("Next State"=w376:T7, "Calibration error?"=w374:bool, "Data out"=w375:T4)  [unwired: 8 in]
        n206 = case shown="False" w374 {
          tunnel: [w384 w386] -> w378
          tunnel: w375 -> [w381 w386]
          frame False {
            # "Calibration image\nloaded succesfully."
            n207 = call "Capture_Save_Initialize.vi"("input cluster"=w381) -> ("output cluster"=w384:T4)  [unwired: 10 in]
            n208 = property on="Stop Image Capture" class="Bool"("DisabledEnum"=T8."Enabled" ("Disabled")) -> ()  [unwired: 2 in, 2 out]
            n209 = property on="Start Image Capture" class="Bool"("DisabledEnum"=T8."Disabled and Grayed Out" ("Disabled")) -> ()  [unwired: 2 in, 2 out]
            n210 = property on="Calibration Pictures" class="Bool"("DisabledEnum"=T8."Disabled and Grayed Out" ("Disabled")) -> ()  [unwired: 2 in, 2 out]
            "Active" <- TRUE ("Image_Capture")
          }
          frame True {
            # "Error loading calibration."
          }
        }
      }
      frame "Stop Image Capture" {
        w388 = T8."Enabled" ("Disabled")
        w391 = FALSE ("Image_Capture")
        w394 = State."Wait for Event"  # Next State
        # "Stop Image Capture\nStopping Camera and Image saving loops."
        n211 = call "Image_Acquisition_Stop.vi"("input cluster"=w390) -> ("output cluster"=w387:T4)  [unwired: 9 in, 1 out]
        n212 = Bundle By Name(cluster=w387, "system.info.captureActive"=w391) -> (w392:T4)
        n213 = local write "Active"(w391) -> ()
        n214 = property on="Start Image Capture" class="Bool"("DisabledEnum"=w388) -> ()  [unwired: 2 in, 2 out]
        n215 = property on="Calibration Pictures" class="Bool"("DisabledEnum"=w388) -> ()  [unwired: 2 in, 2 out]
        n216 = property on="Stop Image Capture" class="Bool"("DisabledEnum"=T8."Disabled and Grayed Out" ("Disabled")) -> ()  [unwired: 2 in, 2 out]
      }
      frame "Calibration Pictures" {
        w396 = TRUE ("Crop?")
        # "Start Image Capture\nTake two calibration pictures with each camera and save in calibration folder."
        n217 = call "Calibration_Capture.vi"("Crop?"=FALSE, "value"=w406) -> ("Image2"=w402:T3, "Image1"=w403:T3, "output cluster"=w410:T4, "error out"=w395:errorcluster)  [unwired: 6 in]
        n218 = case shown="Error .." w395 {
          frame No Error {
          }
          frame Error {
            w414 = T1."Errors" ("Overlay_tab")
            n219 = local write "Overlay_tab"(w414) -> ()
            n220 = local write "Overlay_Ring"(w414) -> ()
          }
        }
        n221 = local write "Camera 2 Detect"(w402) -> ()
        n222 = local write "Camera 1 Detect"(w403) -> ()
        n223 = local write "Errors"(w395) -> ()
        n224 = Unbundle By Name(w406) -> ("system.info.captureBegin"=w407:bool)
        n225 = call "Calibration_Capture.vi"("Detect Movement"=FALSE, "Crop?"=TRUE, "value"=w410) -> ("Image2"=w401:T3, "Image1"=w397:T3, "output cluster"=w398:T4)  [unwired: 5 in, 1 out]
        n226 = local write "Camera 2 Binary"(w401) -> ()
        n227 = local write "Camera 1 Binary"(w397) -> ()
        n228 = call "Calibration_Capture.vi"("Detect Movement"=w396, "Crop?"=w396, "value"=w398) -> ("Image2"=w408:T3, "Image1"=w409:T3, "output cluster"=w404:T4)  [unwired: 5 in, 1 out]
        n229 = case shown="True" w407 {
          tunnel: [w416 w420] -> w413
          tunnel: [w415 w418] -> w405
          tunnel: w404 -> [w415 w417]
          frame False {
            w416 = State."Wait for Event"  # Next State
          }
          frame True {
            w420 = State."Start Image Capture"  # Next State
            n230 = Bundle By Name(cluster=w417, "system.info.captureBegin"=FALSE ("Img_Capt Begin")) -> (w418:T4)
          }
        }
        n231 = local write "Camera 1"(w409) -> ()
        n232 = local write "Camera 2"(w408) -> ()
      }
      frame "Empty and Refill" {
        w435 = T8."Enabled" ("Disabled")
        w433 = TRUE ("Empty_Refill")
        w439 = FALSE ("Image_Capture")
        w443 = State."Valve Signal"  # Next State
        # "Load extra flush volume"
        # "Empty and Refill command\nActivate Empty and refill of cuvette, start listening for valve return signal."
        n233 = Unbundle By Name(w437) -> ("connections.pump.connection"=w428:refnum<visa-resource-name>, "connections.arduino.connection"=w440:refnum<visa-resource-name>, "connections.pump.flushSize"=w421:i32)
        n234 = Number To Decimal String(number=w421) -> (decimal integer string=w424:string)  [unwired: 1 in]
        n235 = Greater Than 0?(x=w421) -> (x > 0?=w422:bool)
        n236 = Concatenate Strings("/1IS20A" ("write buffer 2"), w424, "R" ("string"), "\r\n") -> (w430:string)
        n237 = property on="Empty and Refill" class="Bool"("DisabledEnum"=T8."Disabled and Grayed Out" ("Disabled")) -> ()  [unwired: 2 in, 2 out]
        n238 = property on="Stop Image Capture" class="Bool"("DisabledEnum"=T8."Disabled and Grayed Out" ("Disabled")) -> ()  [unwired: 2 in, 2 out]
        n239 = property on="Start Image Capture" class="Bool"("DisabledEnum"=w435) -> ()  [unwired: 2 in, 2 out]
        n240 = property on="Calibration Pictures" class="Bool"("DisabledEnum"=w435) -> ()  [unwired: 2 in, 2 out]
        n241 = VISA Write(VISA resource name=w440, write buffer="102", error in (no error)=w432) -> (error out=w427:errorcluster)  [unwired: 2 out]
        n242 = case shown="False" w422 {
          tunnel: w430 -> [_ w448]
          tunnel: w428 -> [_ w447]
          tunnel: w427 -> [w444 w446]
          tunnel: [w444 w445] -> w426
          frame False {
          }
          frame True {
            n243 = VISA Write(VISA resource name=w447, write buffer=w448, error in (no error)=w446) -> (error out=w445:errorcluster)  [unwired: 2 out]
          }
        }
        n244 = call "Image_Acquisition_Stop.vi"("input cluster"=w437) -> ("output cluster"=w431:T4)  [unwired: 9 in, 1 out]
        n245 = Tick Count (ms)() -> (millisecond timer value=w434:u32)
        n246 = local write "Active"(w439) -> ()
        n247 = Bundle By Name(cluster=w431, "system.info.captureActive"=w439, "system.info.emptyAndRefill"=w433, "connections.arduino.openState"=w433, "connections.arduino.emptyStart"=w434) -> (w442:T4)
      }
      frame "Close and Refill" {
        w460 = T8."Enabled" ("Disabled")
        w464 = FALSE ("Image_Capture")
        w468 = State."Valve Signal"  # Next State
        # "Empty and Refill command\nActivate Empty and refill of cuvette, start listening for valve return signal."
        n248 = Unbundle By Name(w462) -> ("connections.pump.connection"=w452:refnum<visa-resource-name>, "connections.arduino.connection"=w465:refnum<visa-resource-name>)
        n249 = VISA Write(VISA resource name=w465, write buffer="101", error in (no error)=w457) -> (error out=w451:errorcluster)  [unwired: 2 out]
        n250 = Concatenate Strings("/1IS20A810R" ("write buffer 2"), "\r\n") -> (w455:string)
        n251 = property on="Empty and Refill" class="Bool"("DisabledEnum"=T8."Disabled and Grayed Out" ("Disabled")) -> ()  [unwired: 2 in, 2 out]
        n252 = property on="Stop Image Capture" class="Bool"("DisabledEnum"=T8."Disabled and Grayed Out" ("Disabled")) -> ()  [unwired: 2 in, 2 out]
        n253 = property on="Start Image Capture" class="Bool"("DisabledEnum"=w460) -> ()  [unwired: 2 in, 2 out]
        n254 = property on="Calibration Pictures" class="Bool"("DisabledEnum"=w460) -> ()  [unwired: 2 in, 2 out]
        n255 = VISA Write(VISA resource name=w452, write buffer=w455, error in (no error)=w451) -> (error out=w450:errorcluster)  [unwired: 2 out]
        n256 = call "Image_Acquisition_Stop.vi"("input cluster"=w462) -> ("output cluster"=w456:T4)  [unwired: 9 in, 1 out]
        n257 = Tick Count (ms)() -> (millisecond timer value=w459:u32)
        n258 = local write "Active"(w464) -> ()
        n259 = Bundle By Name(cluster=w456, "system.info.captureActive"=w464, "system.info.emptyAndRefill"=TRUE ("Empty_Refill"), "connections.arduino.openState"=FALSE ("Open(T)/Close(F)"), "connections.arduino.emptyStart"=w459) -> (w467:T4)
      }
      frame "Valve Signal" {
        # "Listen for valve return signal\nListen for valve return signal indicating valve is OPEN or CLOSED."
        n260 = call "Empty_Complete.vi"("input cluster"=w478) -> ("Next State"=w474:T7, "output cluster"=w469:T4)  [unwired: 9 in]
        n261 = local read "Pump"() -> (w470:bool)
        n262 = Equal?(x=State."Pump Cycle" ("Next State"), y=w474) -> (x = y?=w473:bool)
        n263 = Equal?(x=w474, y=State."Wait for Event" ("Next State")) -> (x = y?=w472:bool)
        n264 = Or(x=w473, y=w472) -> (x .or. y?=w471:bool)
        n265 = case shown="True" w471 {
          tunnel: w470 -> [_ w480]
          frame False {
          }
          frame True {
            w479 = T8."Enabled" ("Disabled")
            n266 = case shown="True" w480 {
              frame False {
              }
              frame True {
                n267 = property on="Empty and Refill" class="Bool"("DisabledEnum"=T8."Enabled" ("Disabled")) -> ()  [unwired: 2 in, 2 out]
              }
            }
            n268 = property on="Start Image Capture" class="Bool"("DisabledEnum"=w479) -> ()  [unwired: 2 in, 2 out]
            n269 = property on="Empty Cuvette" class="Bool"("DisabledEnum"=w479) -> ()  [unwired: 2 in, 2 out]
            n270 = property on="Calibration Pictures" class="Bool"("DisabledEnum"=w479) -> ()  [unwired: 2 in, 2 out]
          }
        }
      }
      frame "Position" {
        w491 = State."Wait for Event"  # Next State
        # "Read linear actuator position\nSend command and read linear actuator position."
        n271 = Unbundle By Name(w495) -> ("connections.arduino.connection"=w494:refnum<visa-resource-name>)
        n272 = VISA Write(VISA resource name=w494, write buffer="104", error in (no error)=w492) -> (VISA resource name out=w484:refnum<visa-resource-name>, error out=w490:errorcluster)  [unwired: 1 out]
        n273 = call "Stall Data Flow.vim"("value in"=w484, "milliseconds to wait"=u32 500) -> ("value out"=w482:refnum<visa-resource-name>)  [unwired: 1 out]
        n274 = property class="Instr"(reference=w482, error in=w490) -> (reference out=w488:refnum<visa-resource-name>, error out=w487:errorcluster, "Serial Settings:Number of Bytes at Serial Port"=w489:u32)
        n275 = VISA Read(VISA resource name=w488, byte count=w489, error in (no error)=w487) -> (read buffer=→"Current Position":string, error out=w485:errorcluster)  [unwired: 2 out]
      }
      frame "Valve Cycle" {
        w499 = T8."Enabled" ("Disabled")
        w498 = T8."Disabled and Grayed Out" ("Disabled")
        w502 = FALSE ("Image_Capture")
        w508 = State."Valve Signal"  # Next State
        # "Manual cycle of linear actuator\nRetract and extend linear actuator."
        n276 = Unbundle By Name(w500) -> ("connections.arduino.connection"=w507:refnum<visa-resource-name>)
        n277 = VISA Write(VISA resource name=w507, write buffer="102", error in (no error)=w506) -> (error out=w505:errorcluster)  [unwired: 2 out]
        n278 = property on="Start Image Capture" class="Bool"("DisabledEnum"=w499) -> ()  [unwired: 2 in, 2 out]
        n279 = property on="Calibration Pictures" class="Bool"("DisabledEnum"=w499) -> ()  [unwired: 2 in, 2 out]
        n280 = property on="Stop Image Capture" class="Bool"("DisabledEnum"=w498) -> ()  [unwired: 2 in, 2 out]
        n281 = property on="Empty Cuvette" class="Bool"("DisabledEnum"=w498) -> ()  [unwired: 2 in, 2 out]
        n282 = call "Image_Acquisition_Stop.vi"("input cluster"=w500) -> ("output cluster"=w497:T4)  [unwired: 9 in, 1 out]
        n283 = Tick Count (ms)() -> (millisecond timer value=w503:u32)
        n284 = Bundle By Name(cluster=w497, "connections.arduino.openState"=TRUE ("Open(T)/Close(F)"), "system.info.captureActive"=w502, "system.info.emptyAndRefill"=w502, "connections.arduino.emptyStart"=w503) -> (w501:T4)
      }
      frame "Valve Open" {
        w516 = State."Wait for Event"  # Next State
        w510 = T8."Disabled and Grayed Out" ("Disabled")
        # "Manual extend of linear actuator\nSend extend command to linear actuator."
        n285 = Unbundle By Name(w514) -> ("connections.arduino.connection"=w518:refnum<visa-resource-name>)
        n286 = VISA Write(VISA resource name=w518, write buffer="102", error in (no error)=w519) -> (error out=w517:errorcluster)  [unwired: 2 out]
        n287 = property on="Calibration Pictures" class="Bool"("DisabledEnum"=w510) -> ()  [unwired: 2 in, 2 out]
        n288 = property on="Start Image Capture" class="Bool"("DisabledEnum"=w510) -> ()  [unwired: 2 in, 2 out]
        n289 = property on="Stop Image Capture" class="Bool"("DisabledEnum"=w510) -> ()  [unwired: 2 in, 2 out]
        n290 = call "Image_Acquisition_Stop.vi"("input cluster"=w514) -> ("output cluster"=w512:T4)  [unwired: 9 in, 1 out]
        n291 = Bundle By Name(cluster=w512, "system.info.captureActive"=FALSE ("Image_Capture"), "connections.arduino.openState"=TRUE ("Open(T)/Close(F)")) -> (w511:T4)
      }
      frame "Valve Close" {
        w529 = State."Valve Signal"  # Next State
        # "Manual retract of linear actuator\nSend retract command to linear actuator."
        n292 = Unbundle By Name(w527) -> ("system.info.emptyAndRefill"=w523:bool, "connections.pump.connection"=w521:refnum<visa-resource-name>, "connections.arduino.connection"=w530:refnum<visa-resource-name>)
        n293 = VISA Write(VISA resource name=w530, write buffer="101", error in (no error)=w531) -> (error out=w522:errorcluster)  [unwired: 2 out]
        n294 = case shown="True" w523 {
          tunnel: w522 -> [w532 w538]
          tunnel: w521 -> [_ w537]
          tunnel: [w532 w533] -> w520
          frame False {
            # "Manual Close, don't load volume."
          }
          frame True {
            # "Load specified volume in pump."
            n295 = Concatenate Strings("/1IS20A810R" ("write buffer 2"), "\r\n") -> (w534:string)
            n296 = VISA Write(VISA resource name=w537, write buffer=w534, error in (no error)=w538) -> (error out=w533:errorcluster)  [unwired: 2 out]
          }
        }
        n297 = Tick Count (ms)() -> (millisecond timer value=w525:u32)
        n298 = Bundle By Name(cluster=w527, "connections.arduino.emptyStart"=w525, "connections.arduino.openState"=FALSE ("Open(T)/Close(F)")) -> (w526:T4)
      }
      frame "Pump Command" {
        w547 = State."Wait for Event"  # Next State
        # "<I> Input valve\n<A> Absolute position (n = 1...1000)\n<O> Output valve\n<R> Execute commands\n<T> Abort commands"
        # "Pump command\nSend command to XE 1000 Pump."
        n299 = Unbundle By Name(w546) -> ("connections.pump.connection"=w543:refnum<visa-resource-name>, "connections.pump.command"=w540:string)
        n300 = Concatenate Strings("/1" ("string"), w540, "\r\n") -> (w544:string)
        n301 = VISA Write(VISA resource name=w543, write buffer=w544, error in (no error)=w542) -> (error out=w541:errorcluster)  [unwired: 2 out]
      }
      frame "Pump Cycle" {
        w557 = State."Wait for Event"  # Next State
        # "<I> Input valve\n<A> Absolute position (n = 1...1000)\n<O> Output valve\n<R> Execute commands\n<T> Abort commands"
        # "Pump Cycle\nSend command to XE 1000 Pump going through full cycle."
        n302 = Unbundle By Name(w551) -> ("system.info.emptyAndRefill"=w556:bool, "connections.pump.connection"=w555:refnum<visa-resource-name>, "connections.pump.dispenseSpeed"=w549:i32)
        n303 = Number To Decimal String(number=w549) -> (decimal integer string=w548:string)  [unwired: 1 in]
        n304 = case shown="True" w556 {
          tunnel: w555 -> [w569 w579]
          tunnel: w554 -> [w566 w576]
          tunnel: [w565 w575] -> w553
          tunnel: [u32 3000 ("milliseconds to wait") u32 5000 ("milliseconds to wait")] -> w552
          tunnel: w551 -> [w562 w573]
          tunnel: [w561 w573] -> w550
          tunnel: w548 -> [w559 w571]
          frame True {
            # "Dispense ready volume."
            n305 = Concatenate Strings("/1S" ("write buffer 2"), w559, "OA0R" ("string"), "\r\n") -> (w567:string)
            n306 = Bundle By Name(cluster=w562, "system.info.emptyAndRefill"=FALSE ("Empty_Refill")) -> (w561:T4)
            n307 = VISA Write(VISA resource name=w569, write buffer=w567, error in (no error)=w566) -> (error out=w565:errorcluster)  [unwired: 2 out]
          }
          frame False {
            # "Load and dispense volume."
            n308 = Concatenate Strings("/1IS20A810S" ("write buffer 2"), w571, "OA0R" ("string"), "\r\n") -> (w577:string)
            n309 = VISA Write(VISA resource name=w579, write buffer=w577, error in (no error)=w576) -> (error out=w575:errorcluster)  [unwired: 2 out]
          }
        }
        n310 = Wait (ms)(milliseconds to wait=w552) -> ()  [unwired: 1 out]
      }
      frame "Extra Flush" {
        w587 = State."Valve Close"  # Next State
        # "<I> Input valve\n<A> Absolute position (n = 1...1000)\n<O> Output valve\n<R> Execute commands\n<T> Abort commands"
        # "Pump Extra Flush\nSend command to XE 1000 Pump dispensing an extra flush to clean Cuvette"
        n311 = Unbundle By Name(w586) -> ("connections.pump.connection"=w582:refnum<visa-resource-name>, "connections.pump.dispenseSpeed"=w584:i32)
        n312 = Greater Than 0?(x=w584) -> (x > 0?=w585:bool)
        n313 = Number To Decimal String(number=w584) -> (decimal integer string=w581:string)  [unwired: 1 in]
        n314 = case shown="True" w585 {
          tunnel: w583 -> [w588 w595]
          tunnel: w582 -> [_ w594]
          tunnel: w581 -> [_ w592]
          tunnel: [w588 w589] -> w580
          frame False {
          }
          frame True {
            n315 = Concatenate Strings("/1S" ("write buffer 2"), w592, "OA0R" ("string"), "\r\n") -> (w596:string)
            n316 = VISA Write(VISA resource name=w594, write buffer=w596, error in (no error)=w595) -> (error out=w589:errorcluster)  [unwired: 2 out]
            n317 = Wait (ms)(milliseconds to wait=u32 2000) -> ()  [unwired: 1 out]
          }
        }
      }
      frame "Start System" {
        w609 = State."Empty and Refill"  # Next State
        # "Y<n>: Initialize (Right input, Left output)  (<n> = speed 2-20 sec/stroke)\nS:<n>: Set speed (<n> = 20..600 strokes in 1/10 sec).\nA<n>: Absolute position (<n> = 1...1000)\nI: Input valve\nO: Output valve\nR: Execute commands\nT: Abort commands"
        # "Pump Initialize\nInitialize XE 1000 Pump and fill tubes, emptying cuvette and refill to full."
        n318 = Unbundle By Name(w599) -> ("connections.pump.connection"=w607:refnum<visa-resource-name>)
        n319 = Concatenate Strings("/1Y5IS20A810S60OA0R" ("string"), "\r\n") -> (w608:string)
        n320 = VISA Write(VISA resource name=w607, write buffer=w608, error in (no error)=w606) -> (error out=w605:errorcluster)  [unwired: 2 out]
        n321 = Wait (ms)(milliseconds to wait=u32 10000) -> ()  [unwired: 1 out]
        n322 = Bundle By Name(cluster=w599, "system.info.captureActive"=FALSE ("Img_Capt")) -> (w598:T4)
        n323 = property on="Empty and Refill" class="Bool"("DisabledEnum"=T8."Enabled" ("Disabled")) -> ()  [unwired: 2 in, 2 out]
      }
      frame "Empty System" {
        w627 = State."Valve Cycle"  # Next State
        # "<I> Input valve\n<A> Absolute position (n = 1...1000)\n<O> Output valve\n<R> Execute commands\n<T> Abort commands"
        # "Empty pump and pipes\nSend command to XE 1000 Pump and empty system."
        n324 = Unbundle By Name(w611) -> ("connections.pump.connection"=w625:refnum<visa-resource-name>)
        n325 = Concatenate Strings("/1OS20A1000IA0" ("write buffer 2"), "OS20A1000IA0" ("write buffer 2"), "R" ("write buffer 2")) -> (w620:string)
        n326 = Concatenate Strings(w620, "\r\n") -> (w614:string)
        n327 = VISA Write(VISA resource name=w625, write buffer=w614, error in (no error)=w624) -> (VISA resource name out=w619:refnum<visa-resource-name>, error out=w616:errorcluster)  [unwired: 1 out]
        n328 = property on="Empty and Refill" class="Bool"("DisabledEnum"=T8."Disabled and Grayed Out" ("Disabled")) -> ()  [unwired: 2 in, 2 out]
        n329 = call "Stall Data Flow.vim"("value in"=w619, "milliseconds to wait"=u32 10000) -> ("value out"=w618:refnum<visa-resource-name>)  [unwired: 1 out]
        n330 = VISA Write(VISA resource name=w618, write buffer=w614, error in (no error)=w616) -> (error out=w615:errorcluster)  [unwired: 2 out]
        n331 = Bundle By Name(cluster=w611, "system.info.captureActive"=FALSE ("Img_Capt")) -> (w610:T4)
      }
      frame "CursorIdle" {
        w630 = State."Wait for Event"  # Next State
        # "Manual extend of linear actuator\nSend extend command to linear actuator."
        n332 = call <vilib>:"Unset Busy.vi"("error in (no error)"=w629) -> ("error out"=w628:errorcluster)  [unwired: 10 in]
      }
      frame "Exit" {
        w637 = FALSE ("Pump")
        w639 = FALSE ("Pump")
        w640 = TRUE  # Stop Loop?
        w641 = State."Exit"  # (Value Not Used)
        # "Exit application\nClose all connections, destroy memory allocations, and Exit the application. \n(Potential for saving a settings file)"
        n333 = call "Terminate_Connection.vi"("error in"=w634, "Data"=w636) -> ("error out"=→"error out":errorcluster)  [unwired: 8 in, 1 out]
        n334 = call "Settings_Save.vi"("error in"=w634, "input cluster"=w636) -> ("error out"=w635:errorcluster)  [unwired: 9 in]
        n335 = local write "Active"(w639) -> ()
        n336 = local write "Camera 1"(w639) -> ()
        n337 = local write "Camera 2"(w639) -> ()
        n338 = local write "Pump"(w639) -> ()
        n339 = local write "Actuator"(w639) -> ()
        n340 = Bundle By Name(cluster=w636, "system.info.captureActive"=w637, "connections.arduino.status"=w637, "connections.pump.status"=w637, "connections.camera.cam1.status"=w637, "connections.camera.cam2.status"=w637) -> (w638:T4)
        n341 = property on="Overlay_tab" class="TabCtl (strict)"("Page Labels Display Visible?"=TRUE) -> ()  [unwired: 2 in, 2 out]
      }
    }
    n342 = Or(x=w12, y=FALSE) -> (x .or. y?=w14:bool)
    n343 = call <extravilib>:"Write.vi"("element"=w16) -> ("channel"=w11:T10)  [unwired: 1 out]
    n344 = call <extravilib>:"Write.vi"("element"=w14) -> ("channel"=w10:T11)  [unwired: 1 out]
  }
  n345 = call <vilib>:"Simple Error Handler.vi"("error in (no error)"=w6) -> ("error out"=w5:errorcluster)  [unwired: 4 in, 4 out]
  n346 = disable-structure shown="RUN_TIME_ENGINE==True" {
    disable-tunnel: w5 -> [_ _]
    frame condition #0 (active) {
    }
    frame condition #1 {
      # "Call Quit LabVIEW if running as a built application."
      n347 = Quit LabVIEW() -> ()  [unwired: 1 in]
    }
  }
  n348 = while {
    tunnel: w3 -> [w643]
    tunnel: w2 -> [w647]
    tunnel: [w642] -> w1
    stop <- w649 stop-if-true
    # "Image handling - object detection"
    n349 = call <extravilib>:"Read.vi"("channel"=w647) -> ("element"=w645:T4)  [unwired: 1 in, 1 out]
    n350 = Unbundle By Name(w645) -> ("system.info.captureActive"=w646:bool)
    n351 = case shown="True" w646 {
      tunnel: [TRUE ("Last Image?") w658] -> w648
      tunnel: w647 -> [_ w659]
      tunnel: [w652 w657] -> w642
      frame False {
        # "Image capture inactive"
        n352 = Bundle(TRUE, FALSE) -> (w653:cluster{bool, bool})  [unwired: 1 in]
        n353 = call <extravilib>:"Write.vi"("element"=w653) -> ("channel"=w652:T12)  [unwired: 1 out]
        n354 = local write "Process buffer"(T2 {"# elements in queue"=0, "# elements in queue"=0} ("Image processing")) -> ()
        n355 = Wait (ms)(milliseconds to wait=u32 10) -> ()  [unwired: 1 out]
      }
      frame True {
        # "Image capture active"
        n356 = while "Save image" {
          tunnel: w659 -> [w666]
          tunnel: [w667] -> w658
          tunnel: [w661] -> w657
          stop <- w667 stop-if-true
          # "Image Processing"
          n357 = call <extravilib>:"Read.vi"("channel"=w666) -> ("element"=w665:T4)  [unwired: 1 in, 1 out]
          n358 = call "Image_Processing_Queue.vi"("Data"=w665) -> ("Status"=w661:T12, "Detection error"=→"Detection error":errorcluster, "Process queue"=→"Process buffer":T2, "Last Image?"=w667:bool, "Image 1"=→"Camera 1":T3, "Image 2"=→"Camera 2":T3, "Binary 1"=→"Camera 1 Binary":T3, "Binary 2"=→"Camera 2 Binary":T3)  [unwired: 9 in, 2 out]
        }
      }
    }
    n359 = call <extravilib>:"Read.vi"("channel"=w643) -> ("element"=w644:bool)  [unwired: 1 in, 1 out]
    n360 = And(x=w648, y=w644) -> (x .and. y?=w649:bool)
  }
  n361 = while {
    tunnel: w3 -> [w680]
    tunnel: w2 -> [w679]
    tunnel: w1 -> [w673]
    stop <- w677 stop-if-true
    # "Camera Handler"
    n362 = call <extravilib>:"Read.vi"("channel"=w673) -> ("element"=w672:cluster{bool, bool})  [unwired: 1 in, 1 out]
    n363 = call <extravilib>:"Read.vi"("channel"=w679) -> ("element"=w678:T4)  [unwired: 1 in, 1 out]
    n364 = Unbundle(w672) -> (w670:bool, w671:bool)
    n365 = Unbundle By Name(w678) -> ("system.info.captureActive"=w675:bool)
    n366 = call <extravilib>:"Read.vi"("channel"=w680) -> ("element"=w677:bool)  [unwired: 1 in, 1 out]
    n367 = Not(x=w671) -> (.not. x?=w676:bool)
    n368 = And(x=w676, y=w675) -> (x .and. y?=w674:bool)
    n369 = case shown="True" w674 {
      tunnel: w678 -> [_ w684]
      tunnel: w670 -> [_ w683]
      frame False {
        # "Empty Case\nImage Capture currently inactive."
        n370 = local write "Framerate"(0.0 ("Framerate")) -> ()
        n371 = Wait (ms)(milliseconds to wait=u32 20) -> ()  [unwired: 1 out]
      }
      frame True {
        # "Capture Image\nImage Capture currently active, transmitting data."
        n372 = call "Image_Snap_Dual.vi"("input cluster"=w684, "Detect Movement"=w683) -> ("Framerate"=→"Framerate":i32)  [unwired: 6 in, 3 out]
      }
    }
  }
  n373 = while {
    tunnel: w2 -> [w690]
    tunnel: w3 -> [w688]
    tunnel: w2 -> [w686]
    stop <- w692 stop-if-true
    # "Image Save"
    n374 = call <extravilib>:"Read.vi"("channel"=w690) -> ("element"=w689:T4)  [unwired: 1 in, 1 out]
    n375 = call <extravilib>:"Read.vi"("channel"=w688) -> ("element"=w691:bool)  [unwired: 1 in, 1 out]
    n376 = Unbundle By Name(w689) -> ("system.info.captureActive"=w693:bool)
    n377 = case shown="True" w693 {
      selector: w693 -> [_ w698]
      tunnel: w688 -> [_ w701]
      tunnel: [TRUE ("Last Image?") w699] -> w687
      tunnel: w686 -> [_ w700]
      frame False {
        n378 = local write "Save buffer"(T2 {"# elements in queue"=0, "# elements in queue"=0} ("Image Saving")) -> ()
        n379 = Wait (ms)(milliseconds to wait=u32 10) -> ()  [unwired: 1 out]
      }
      frame True {
        n380 = while {
          tunnel: w701 -> [w715]
          tunnel: w700 -> [w714]
          tunnel: [w711] -> w699
          shift-right: [FALSE] -> _
          shift-left: w698 -> [w707]
          stop <- w711 stop-if-true
          n381 = call <extravilib>:"Read.vi"("channel"=w714) -> ("element"=w713:T4)  [unwired: 1 in, 1 out]
          n382 = call <extravilib>:"Read.vi"("channel"=w715) -> ("element"=w712:bool)  [unwired: 1 in, 1 out]
          n383 = call "Image_Save_Handler.vi"("first iteration"=w707, "Data"=w713, "Stop?"=w712) -> ("Image Save 1"=→"Camera 1 Detect":T3, "Image Save 2"=→"Camera 2 Detect":T3, "Cam2_Stats"=→"Cam2_Stats":cluster{"Mean_Area":i32, "Img_Count":u32}, "Cam1_Stats"=→"Cam1_Stats":cluster{"Mean_Area":i32, "Img_Count":u32}, "Queue size"=→"Save buffer":T2, "timeout"=→"Ready":bool, "Sample Name"=→"Sample Number":string, "Stop out"=w711:bool)  [unwired: 16 in, 1 out]
        }
      }
    }
    n384 = And(x=w687, y=w691) -> (x .and. y?=w692:bool)
    n385 = case shown="True" w692 {
      frame False {
      }
      frame True {
        n386 = call "IMAQ Dispose"("All Images? (No)"=TRUE) -> ()  [unwired: 5 in, 1 out]
      }
    }
  }
